vi "XIPIN_3GPP_LTE_MIMO_Encoder_2_0.vi"   [LabVIEW 2017]
doc: "The LTE 3GPP MIMO Encoder v2.0 core implements multiple-input, multiple-output (MIMO) encoding for LTE eNodeB applications as defined in the 3GPP TS 36.211 specification.\n------------------------------------\n<b>Need License</b> : Yes"
uses:
  <vilib>/rvi/XilinxIP/XIPIN_XNode/niFpgaXIPIN.xnode
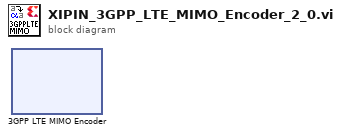
[diagram p0: block diagram]
diagram:
  n1 = xnode ("3GPP LTE MIMO Encoder")() -> ()
